vi "Init Paths.vi"(8 "Error In":errorcluster, 11 "WebView in":refnum<class "WebView.lvclass">) -> (0 "Error Out":errorcluster, 3 "WebView out":refnum<class "WebView.lvclass">)   [LabVIEW 2024, in "WebView.lvclass"]
uses:
  WebView.lvclass
  Paths-cluster.ctl
  <vilib>/Utility/sysdir.llb/System Directory Type.ctl
  WebView.lvclass/WebView.ctl
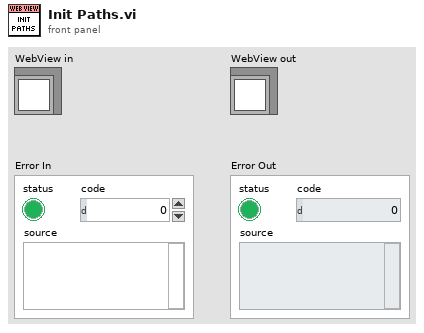
[diagram p1: front panel]
types:
  T1 = typedef "System Directory Type.ctl" = i32
  T2 = typedef "WebView.lvclass/Paths-cluster.ctl" = cluster{"Webview2 Native":path, "Edge Application":path, "User Data":path}
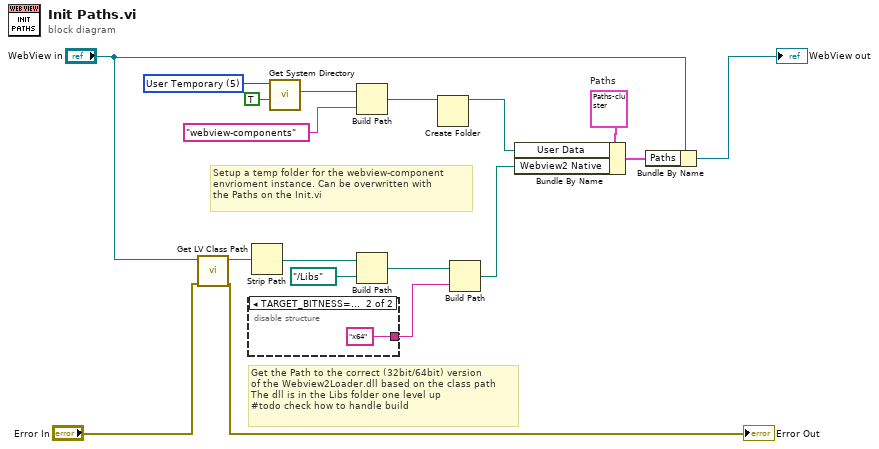
[diagram p0: block diagram]
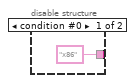
[diagram p2: hidden frame]
diagram:
  w15 = T1 5 items=["User Home"=0, "User Desktop"=1, "User Documents"=2, "User Application Data"=3, "User Preferences"=4, "User Temporary"=5, "Public Documents"=6, "Public Application Data"=7, "Public Preferences"=8, "Public Cache"=13, "System Core Libraries"=9, "System Installed Libraries"=10, "Application Files"=11, "Boot Volume Root"=12] ("system directory type")
  w17 = T2 {"Webview2 Native"=path "C:/Users/kleins/Desktop/webview2/microsoft.web.webview2.1.0.1370.28/build/native", "Edge Application"=path "", "User Data"=path ""}  # Paths
  # "Setup a temp folder for the webview-component\nenvrioment instance. Can be overwritten with \nthe Paths on the Init.vi"
  # "Get the Path to the correct (32bit/64bit) version \nof the Webview2Loader.dll based on the class path\nThe dll is in the Libs folder one level up\n#todo check how to handle build"
  n1 = call <vilib>:"Get LV Class Path.vi"("error in (no error)"="Error In", "object"="WebView in") -> ("error out"=→"Error Out":errorcluster, "class path"=w7:path)  [unwired: 8 in]
  n2 = disable-structure shown="TARGET_BITNESS==64" {
    disable-tunnel: ["x86" "x64"] -> w11
    frame condition #0 {
    }
    frame condition #1 (active) {
    }
  }
  n3 = Strip Path(path=w7) -> (stripped path=w4:path)  [unwired: 1 out]
  n4 = call <vilib>:"Get System Directory.vi"("create directory if not found? (F)"=TRUE, "system directory type"=w15) -> ("system directory"=w14:path)  [unwired: 9 in]
  n5 = Build Path(base path=w14, name or relative path="webview-components") -> (appended path=w2:path)
  n6 = Build Path(base path=w4, name or relative path=path "../Libs") -> (appended path=w10:path)
  n7 = Create Folder(path (use dialog)=w2) -> (created path=w1:path)  [unwired: 2 in, 2 out]
  n8 = Build Path(base path=w10, name or relative path=w11) -> (appended path=w9:path)
  n9 = Bundle By Name(cluster=w17, "User Data"=w1, "Webview2 Native"=w9) -> (w16:T2)
  n10 = Bundle By Name(cluster="WebView in", "Paths"=w16) -> (→"WebView out":refnum<class "WebView.lvclass">)
